vi "Constant getFileTitle.vi"(3 "Enum":T1(ring)) -> (0 "List Param String":string, 1 "List Params Array":string[](array[string]))   [LabVIEW 2018]
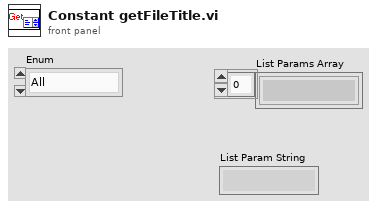
[diagram p1: front panel]
types:
  T1 = enum16{"All", "Path", "Time Stamp", "Group Name", "File Name", "Retention Time", "Param1"}
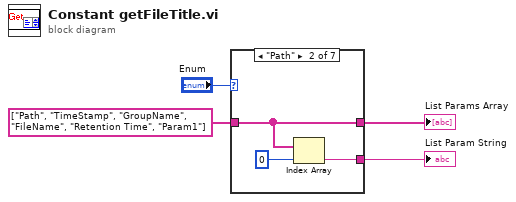
[diagram p0: block diagram]
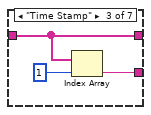
[diagram p3: hidden frame]
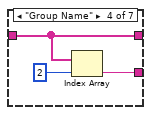
[diagram p4: hidden frame]
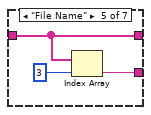
[diagram p5: hidden frame]
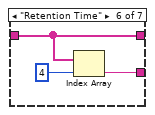
[diagram p6: hidden frame]
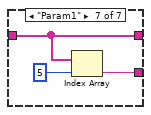
[diagram p7: hidden frame]
diagram:
  n1 = case shown="\"Path\"" "Enum" {
    tunnel: string[] ["Path", "TimeStamp", "GroupName", "FileName", "Retention Time", "Param1"] ("List Param Array") -> [w5 w6 w9 w12 w15 w18 w21]
    tunnel: [w5 w6 w9 w12 w15 w18 w21] -> w2
    tunnel: [_ w7 w10 w13 w16 w19 w22] -> w1
    frame "All", Default {
    }
    frame "Path" {
      n2 = Index Array(array=w6, index=0) -> (element=w7:string)
    }
    frame "Time Stamp" {
      n3 = Index Array(array=w9, index=1) -> (element=w10:string)
    }
    frame "Group Name" {
      n4 = Index Array(array=w12, index=2) -> (element=w13:string)
    }
    frame "File Name" {
      n5 = Index Array(array=w15, index=3) -> (element=w16:string)
    }
    frame "Retention Time" {
      n6 = Index Array(array=w18, index=4) -> (element=w19:string)
    }
    frame "Param1" {
      n7 = Index Array(array=w21, index=5) -> (element=w22:string)
    }
  }
  "List Params Array" <- w2
  "List Param String" <- w1
